vi "08-send-and-receive-img.vi"() -> ()   [LabVIEW 2018, in "LV-0mq-Julia_roundtrip-lib.lvlib"]
uses:
  LV-0mq-Julia_roundtrip-lib.lvlib
  Server or client state.ctl
  Commands.ctl
  f9264f0d-2c2d-4a22-a0da-9e005a3dfb77.vi
  f9264f0d-2c2d-4a22-a0da-9e005a3dfb77.vi/7e17abd8-931d-48a1-8db6-a024c53a6638.vi
  f9264f0d-2c2d-4a22-a0da-9e005a3dfb77.vi/7e17abd8-931d-48a1-8db6-a024c53a6638.vi/903c1eda-13a4-480e-b97e-2d0b6d028f08.vi
  f9264f0d-2c2d-4a22-a0da-9e005a3dfb77.vi/7e17abd8-931d-48a1-8db6-a024c53a6638.vi/07d0fb82-edb9-498c-83ef-1030a08e46c3.vi
  f9264f0d-2c2d-4a22-a0da-9e005a3dfb77.vi/7e17abd8-931d-48a1-8db6-a024c53a6638.vi/8611fb42-f52c-4cb5-8724-17158622ca55.vi
  jl-scripts path.vi
  <vilib>/Utility/error.llb/Error Cluster From Error Code.vi
  check ID validity.vi
  bindata_descr to JSON.vi
  check cluster field names.vi
  concat JSON.vi
  build request.vi
  Parse server response.vi
  log jl exceptions.vi
  <vilib>/ErrorRing/Error Ring.xnode
panel:
  in  "Transform":T1
  out "picture sent":picture
  in  "image file path":path=path "../other_files/peppers_color_256.png"
  out "picture received":picture
  out "short error info":string
  in  "next":bool
  out "current error":errorcluster
  out "final error":errorcluster
  in  "stop":bool
  out "ZMQ timeout":bool
  out "Julia script file path":path
  out "temporary script path":path
  out "Jl Server state":T2
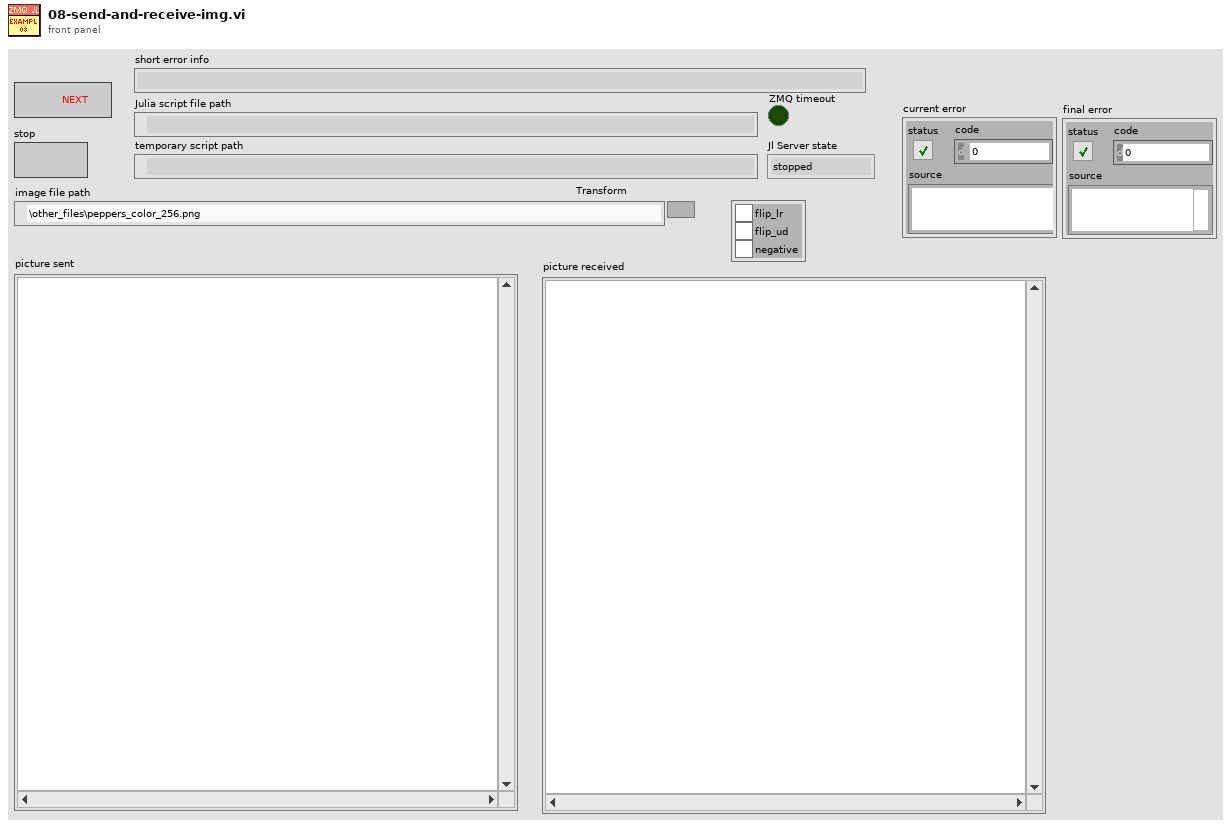
[diagram p1: front panel]
types:
  T1 = cluster{"flip_lr":bool, "flip_ud":bool, "negative":bool}
  T2 = typedef "LV-0mq-Julia_roundtrip-lib.lvlib/Server or client state.ctl" = enum16{"stopped", "running", "unknown"}
  T3 = typedef "LV-0mq-Julia_roundtrip-lib.lvlib/Commands.ctl" = enum16{"Start Jl-server & Init LV-client", "Send request & Get response ", "Stop Jl-server & Cleanup LV-client", "Cleanup LV-client", "Start Jl-server", "Stop Jl-server", "Init LV-Client", "Cleanup LV-Client", "(not allowed)", "Set LV Client state", "Set Jl Server state", "set ZMQ timeout", "read ZMQ timeout", "read-out state"}
  T4 = typedef "imagedata.ctl" = cluster{"image type":i32, "image depth":i32, "image":u8[], "mask":u8[], "colors":u32[], "Rectangle":cluster{"left":i16, "top":i16, "right":i16, "bottom":i16}}
  T5 = typedef "LV-0mq-Julia_roundtrip-lib.lvlib/Bindata&description.ctl" = cluster{"bindata_descr":T6[], "bindata":u8[]}
  T6 = typedef "LV-0mq-Julia_roundtrip-lib.lvlib/Bindata description.ctl" = cluster{"nofbytes":i32, "numtype":string, "start":i32, "arrdims":i32[], "kwarg_name":string, "category":string}
  T7 = typedef "LV-0mq-Julia_roundtrip-lib.lvlib/detailed error info.ctl" = cluster{"exception_or_info":string, "trace":T8[]}
  T8 = typedef "LV-0mq-Julia_roundtrip-lib.lvlib/StackFrame.ctl" = cluster{"frame_summary":string, "func":string, "linfo":string, "file":string, "line":i32, "pointer":u64, "from_c":bool, "inlined":bool}
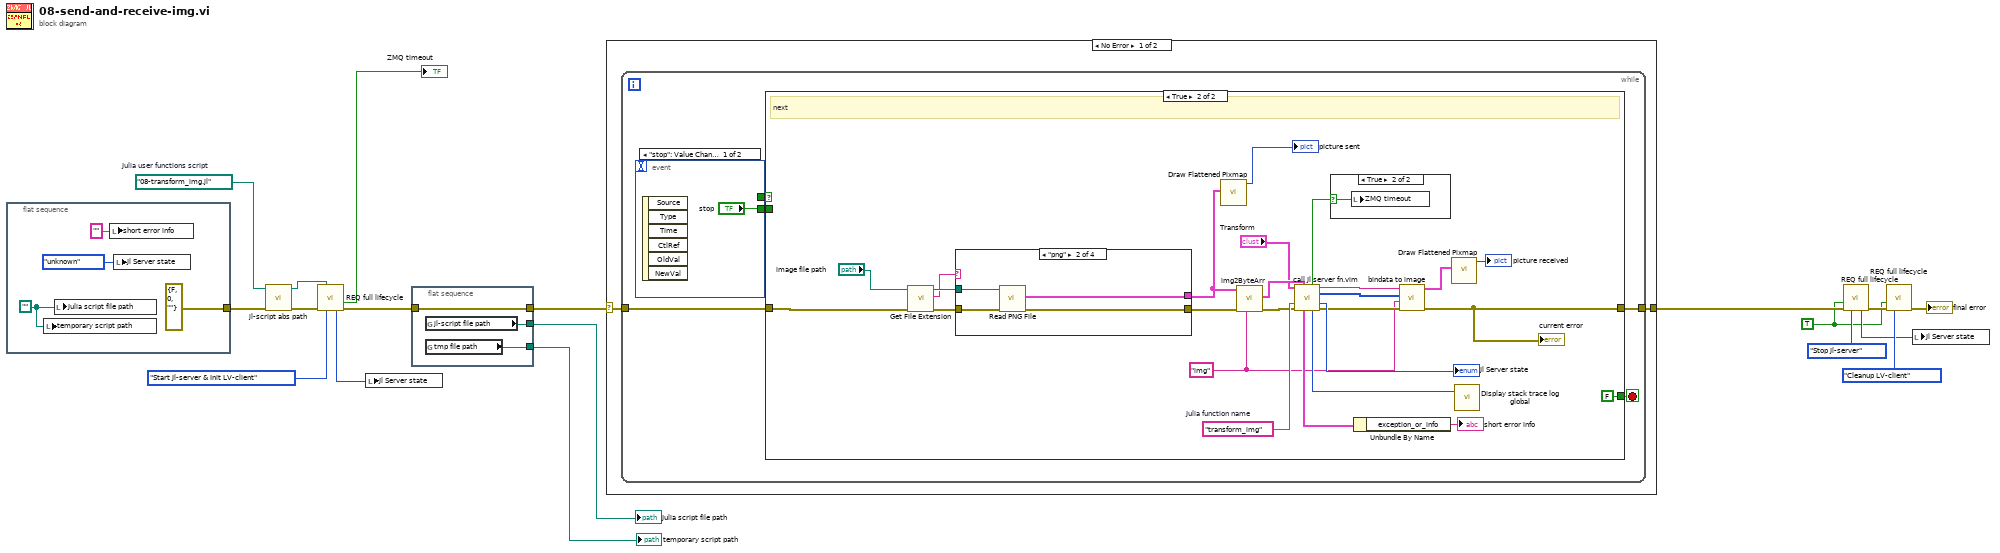
[diagram p0: block diagram]
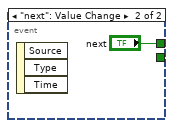
[diagram p2: hidden frame]
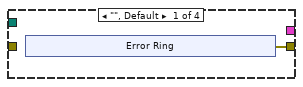
[diagram p4: hidden frame]
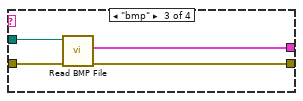
[diagram p5: hidden frame]
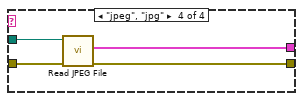
[diagram p6: hidden frame]
diagram:
  w5 = path "08-transform_img.jl"  # Julia user functions script
  w2 = TRUE ("Force command")
  n1 = flat-sequence {
    tunnel: [errorcluster {"status"=FALSE, "code"=0, "source"=""} ("error in (no error)")] -> w3
    frame #0 {
      w20 = path ""
      n2 = local write "temporary script path"(w20) -> ()
      n3 = local write "Julia script file path"(w20) -> ()
      n4 = local write "short error info"("" ("short error info")) -> ()
      n5 = local write "Jl Server state"(Server_or_client_state."unknown" ("Jl Server state out")) -> ()
    }
  }
  n6 = call "jl-script abs path.vi"("error in (no error)"=w3, "Julia user functions script"=w5) -> ("error out"=w6:errorcluster, "script abs path"=w7:path)  [unwired: 8 in]
  n7 = call "REQ full lifecycle.vi"("Julia user functions script"=w7, "error in"=w6, "command"=Commands."Start Jl-server & Init LV-client") -> ("timeout?"=→"ZMQ timeout":bool, "Jl Server state out"=w8:T2, "error out"=w1:errorcluster)  [unwired: 6 in, 4 out]
  n8 = local write "Jl Server state"(w8) -> ()
  n9 = flat-sequence {
    tunnel: [w25] -> w13
    tunnel: w1 -> [w25]
    tunnel: [w24] -> w11
    tunnel: [w23] -> w12
    frame #0 {
      n10 = global read "jl-scripts path.vi" "jl-script file path"() -> (w24:path)
      n11 = global read "jl-scripts path.vi" "tmp file path"() -> (w23:path)
    }
  }
  n12 = case shown="No Error" w13 {
    selector: w13 -> [w26 w81]
    tunnel: [w27 w81] -> w18
    frame No Error {
      n13 = while {
        tunnel: w26 -> [w31]
        tunnel: [w32] -> w27
        stop <- w29 stop-if-true
        n14 = event shown="[0] \"stop\": Value Change" {
          selector: _ -> [_ _]
          dyn-events: _ -> [_ _]
          timeout: _ -> [_ _]
          tunnel: [_ "next"] -> w30
          tunnel: ["stop" _] -> w28
          event "stop": Value Change {
            n15 = event-data() -> ()  [unwired: 1 in, 6 out]
          }
          event "next": Value Change {
            n16 = event-data() -> ()  [unwired: 1 in, 3 out]
          }
        }
        n17 = case shown="True" w30 {
          tunnel: [w36 w51] -> w32
          tunnel: w31 -> [w36 w42]
          tunnel: [w35 FALSE ("stop this VI only")] -> w29
          tunnel: w28 -> [w35 _]
          frame False {
            # "stop"
          }
          frame True {
            w40 = "img" ("name")
            w60 = "transform_img"  # Julia function name
            # "next"
            n18 = call <vilib>:"Get File Extension.vi"("error in (no error)"=w42, "file"="image file path") -> ("error out"=w45:errorcluster, "lowercase file extension"=w43:string, "dup file"=w46:path)  [unwired: 5 in, 2 out]
            n19 = case shown="\"png\"" w43 {
              tunnel: [_ w71 w75 w79] -> w48
              tunnel: w46 -> [_ w70 w74 w78]
              tunnel: w45 -> [_ w69 w73 w77]
              tunnel: [w62 w68 w72 w76] -> w44
              frame "", Default {
                n20 = xnode "Error Ring"() -> ("error out"=w62:errorcluster)
              }
              frame "png" {
                n21 = call <vilib>:"Read PNG File.vi"("error in (no error)"=w69, "path to PNG file"=w70) -> ("error out"=w68:errorcluster, "image data"=w71:T4)  [unwired: 7 in, 1 out]
              }
              frame "bmp" {
                n22 = call <vilib>:"Read BMP File.vi"("error in (no error)"=w73, "path to BMP file"=w74) -> ("error out"=w72:errorcluster, "image data"=w75:T4)  [unwired: 7 in, 1 out]
              }
              frame "jpeg", "jpg" {
                n23 = call <vilib>:"Read JPEG File.vi"("error in (no error)"=w77, "path to JPEG file"=w78) -> ("error out"=w76:errorcluster, "image data"=w79:T4)  [unwired: 7 in, 1 out]
              }
            }
            n24 = call <vilib>:"Draw Flattened Pixmap.vi"("image data"=w48) -> ("new picture"=→"picture sent":picture)  [unwired: 8 in]
            n25 = call "img2ByteArr.vi"("kwarg_name"=w40, "error in (no error)"=w44, "img in"=w48) -> ("error out"=w41:errorcluster, "Bindata & descr out"=w38:T5)  [unwired: 6 in, 1 out]
            n26 = call "call Jl server fn.vim"("Arguments 1"="Transform", "Bindata & descr in"=w38, "fun2call"=w60, "error in (no error)"=w41) -> ("timeout?"=w58:bool, "JSON received"=w50:string, "binary data received"=w49:u8[], "Jl Server state out"=→"Jl Server state":T2, "detailed error info"=w56:T7, "return code"=w57:u8, "error out"=w52:errorcluster)  [unwired: 5 in]
            n27 = case shown="True" w58 {
              selector: w58 -> [_ w80]
              frame False {
              }
              frame True {
                n28 = local write "ZMQ timeout"(w80) -> ()
              }
            }
            n29 = Unbundle By Name(w56) -> ("exception_or_info"=→"short error info":string)
            n30 = call "bindata to image.vi"("error in (no error)"=w52, "name"=w40, "binary data in"=w49, "JSON in"=w50) -> ("error out"=w51:errorcluster, "img out"=w53:T4)  [unwired: 6 in]
            "current error" <- w51
            n31 = call <vilib>:"Draw Flattened Pixmap.vi"("image data"=w53) -> ("new picture"=→"picture received":picture)  [unwired: 8 in]
            n32 = call "Display stack trace log global.vi"("return code"=w57) -> ()  [unwired: 3 in]
          }
        }
      }
    }
    frame Error {
    }
  }
  n33 = call "REQ full lifecycle.vi"("Force command"=w2, "error in"=w18, "command"=Commands."Stop Jl-server") -> ("Jl Server state out"=w10:T2, "error out"=w16:errorcluster)  [unwired: 6 in, 5 out]
  n34 = call "REQ full lifecycle.vi"("Force command"=w2, "error in"=w16, "command"=Commands."Cleanup LV-client") -> ("error out"=→"final error":errorcluster)  [unwired: 6 in, 6 out]
  n35 = local write "Jl Server state"(w10) -> ()
  "temporary script path" <- w12
  "Julia script file path" <- w11
